vi "BrakeFail.vi"(8 "error in (no error)":errorcluster, 10 "Cluster in":T1, 11 "Enum in":T2) -> (0 "error out":errorcluster, 2 "Cluster":T1, 3 "Enum out":T2)   [LabVIEW 2018]
uses:
  Type_Def/Type_Def ControlState.ctl
  Type_Def/Type_Def Actuator Controls.ctl
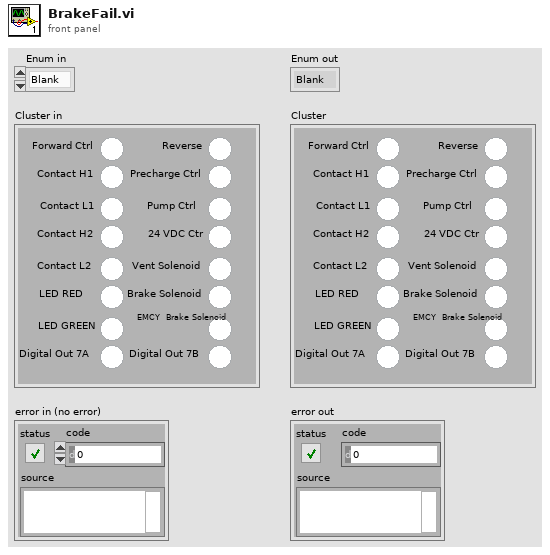
[diagram p1: front panel]
types:
  T1 = typedef "Type_Def Actuator Controls.ctl" = cluster{"Reverse ":bool, "Precharge Ctrl":bool, "Pump Ctrl":bool, "24 VDC Ctr":bool, "Vent Solenoid":bool, "Brake Solenoid":bool, "EMCY  Brake Solenoid":bool, "Digital Out 7B ":bool, "Forward Ctrl":bool, "Contact H1":bool, "Contact L1":bool, "Contact H2":bool, "Contact L2 ":bool, "LED RED":bool, "LED GREEN":bool, " Digital Out 7A":bool}
  T2 = typedef "Type_Def ControlState.ctl" = enum16{"Blank", "Systems Check", "Idle", "Ready", "Pushing", "CrawlingPrecharge", "Braking", "Fault", "Boot Up", "Unpowered", "Crawling", "Shutdown", "Service Push", "Service Wait", "Vent", "Precharge"}
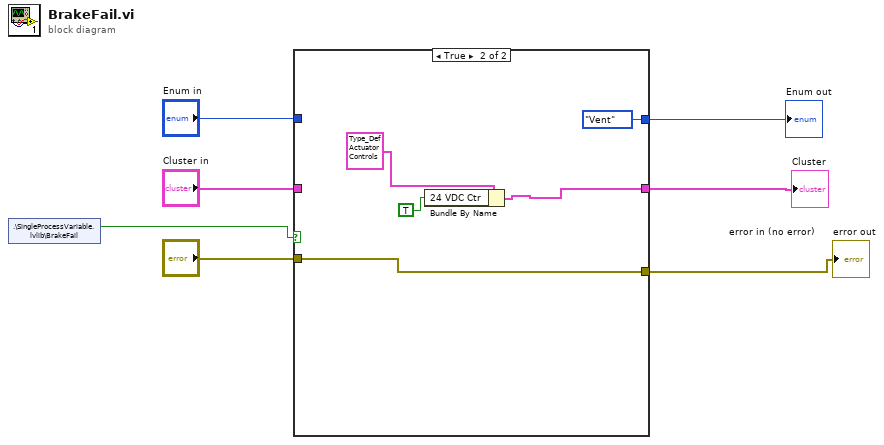
[diagram p0: block diagram]
diagram:
  n1 = shared-variable ".\\SingleProcessVariable.lvlib\\BrakeFail"() -> (w1:bool)  [unwired: 1 in, 1 out]
  n2 = case shown="True" w1 {
    tunnel: [w8 w15] -> w7
    tunnel: "error in (no error)" -> [w8 w15]
    tunnel: [w9 w11] -> w5
    tunnel: "Cluster in" -> [w9 _]
    tunnel: [w10 Type_Def_ControlState."Vent" ("Enum in")] -> w3
    tunnel: "Enum in" -> [w10 _]
    frame False {
    }
    frame True {
      n3 = Bundle By Name(cluster=T1 {"Reverse "=FALSE, "Precharge Ctrl"=FALSE, "Pump Ctrl"=FALSE, "24 VDC Ctr"=FALSE, "Vent Solenoid"=FALSE, "Brake Solenoid"=FALSE, "EMCY  Brake Solenoid"=FALSE, "Digital Out 7B "=FALSE, "Forward Ctrl"=FALSE, "Contact H1"=FALSE, "Contact L1"=FALSE, "Contact H2"=FALSE, "Contact L2 "=FALSE, "LED RED"=FALSE, "LED GREEN"=FALSE, " Digital Out 7A"=FALSE} ("Cluster in 2"), "24 VDC Ctr"=TRUE) -> (w11:T1)
    }
  }
  "Enum out" <- w3
  "error out" <- w7
  "Cluster" <- w5
